vi "CreatePadNode.vi"(8 "Error In":errorcluster, 10 "Pad Number":u32, 11 "DOM Document":refnum<k20>) -> (0 "Error Out":errorcluster, 3 "Pad Element":refnum<k20>)   [LabVIEW 2012, in "Virtual-PGA.lvlib"]
uses:
  Virtual-PGA.lvlib
  <resource>/objmgr/DOMUserDefRef.rc
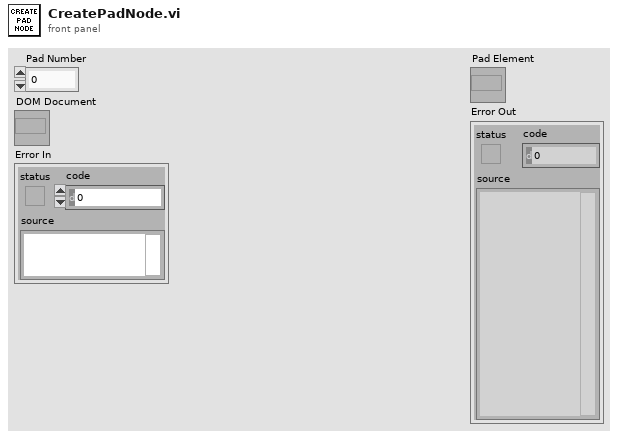
[diagram p1: front panel]
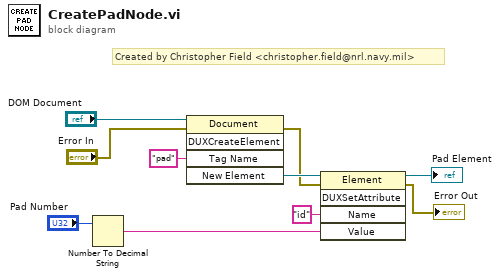
[diagram p0: block diagram]
diagram:
  # "Created by Christopher Field <christopher.field@nrl.navy.mil>"
  n1 = Number To Decimal String(number="Pad Number") -> (decimal integer string=w7:string)  [unwired: 1 in]
  n2 = invoke class="Document" method="DUXCreateElement"(reference="DOM Document", error in="Error In", "Tag Name"="pad") -> (error out=w6:errorcluster, "New Element"=w9:refnum<k20>)  [unwired: 2 in, 3 out]
  n3 = invoke class="Element" method="DUXSetAttribute"(reference=w9, error in=w6, "Name"="id", "Value"=w7) -> (reference out=→"Pad Element":refnum<k20>, error out=→"Error Out":errorcluster)  [unwired: 1 in, 3 out]
